vi "Unset Cursor.vi"(8 "error in (no error)":errorcluster, 11 "Cursor in":refnum<class "Cursor.lvclass">) -> (0 "error out":errorcluster)   [LabVIEW 2019, in "Panel.lvlib" / "Cursor.lvclass"]
doc: "Unsets the cursor busy if the Control Counter is fully released.\n\n----\nPlease see the following web address for additional documentation and tutorial information:\nhttp://www.mooregoodideas.com/mgi-panel-manager/\n\nAuthor: Derek Trepanier\n\nCopyright (c) 2018, Moore Good Ideas, Inc.\n\nAll rights reserved.\n\nRedistribution and use in source and binary forms, with or without modification, are permitted provided that the following conditions are met:\n\n * Redistributions of source code must retain the above copyright notice, this list of conditions and the following disclaimer.\n * Redistributions in binary form must reproduce the above copyright notice, this list of conditions and the following disclaimer in the documentation and/or other materials provided with the distribution.\n * Neither the name of Moore Good Ideas, Inc. nor the names of its contributors may be used to endorse or promote products derived from this software without specific prior written permission.\n\nTHIS SOFTWARE IS PROVIDED BY THE COPYRIGHT HOLDERS AND CONTRIBUTORS \"AS IS\" AND ANY EXPRESS OR IMPLIED WARRANTIES, INCLUDING, BUT NOT LIMITED TO, THE IMPLIED WARRANTIES OF MERCHANTABILITY AND FITNESS FOR A PARTICULAR PURPOSE ARE DISCLAIMED. IN NO EVENT SHALL THE COPYRIGHT OWNER OR CONTRIBUTORS BE LIABLE FOR ANY DIRECT, INDIRECT, INCIDENTAL, SPECIAL, EXEMPLARY, OR CONSEQUENTIAL DAMAGES (INCLUDING, BUT NOT LIMITED TO, PROCUREMENT OF SUBSTITUTE GOODS OR SERVICES; LOSS OF USE, DATA, OR PROFITS; OR BUSINESS INTERRUPTION) HOWEVER CAUSED AND ON ANY THEORY OF LIABILITY, WHETHER IN CONTRACT, STRICT LIABILITY, OR TORT (INCLUDING NEGLIGENCE OR OTHERWISE) ARISING IN ANY WAY OUT OF THE USE OF THIS SOFTWARE, EVEN IF ADVISED OF THE POSSIBILITY OF SUCH DAMAGE."
uses:
  Cursor.lvclass
  Cursor.lvclass/Cursor.ctl
  Panel Control Counter/Panel Control Counter.lvclass
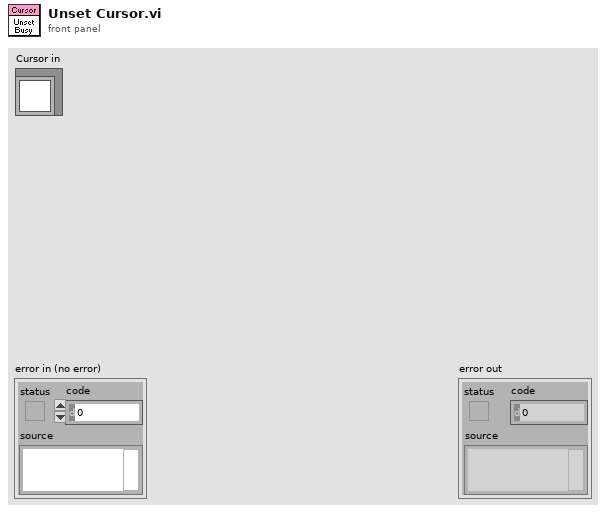
[diagram p1: front panel]
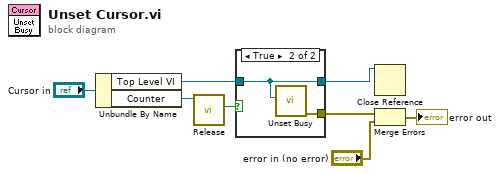
[diagram p0: block diagram]
diagram:
  n1 = Unbundle By Name("Cursor in") -> ("Top Level VI"=w4:refnum<vi>, "Counter"=w6:refnum<class "Panel Control Counter.lvclass">)
  n2 = call "Release.vi"("Panel Control Counter in"=w6) -> ("Fully Released?"=w5:bool)  [unwired: 9 in, 1 out]
  n3 = case shown="True" w5 {
    tunnel: w4 -> [w9 w10]
    tunnel: [_ w11] -> w2
    tunnel: [w9 w10] -> w1
    frame False {
    }
    frame True {
      n4 = call <vilib>:"Unset Busy.vi"("VI reference (current VI)"=w10) -> ("error out"=w11:errorcluster)  [unwired: 10 in]
    }
  }
  n5 = Close Reference(reference=w1) -> ()  [unwired: 1 in, 1 out]
  n6 = Merge Errors(w2, "error in (no error)") -> (→"error out":errorcluster)
